vi "Convert Package Display Name (VIPM to NIPM).vi"(8 "error in (no error)":errorcluster, 9 "LabVIEW version in":string, 11 "VIPM Package Display Name":string) -> (0 "error out":errorcluster, 1 "LabVIEW version out":string, 3 "NIPM Package Display Name":string)   [LabVIEW 2014, in "vipm-to-nipm-package-converter.lvlib"]
doc: "Converts the VIPM package's Display Name to a LabVIEW-version specific NIPM Package Display Name. For example, \"OpenG String Library\" and \"18.0\" converts to \"OpenG String Library (LabVIEW 2018 32-bit)\".\n\nINPUT(S):\n<b>LabVIEW version</b>: Specifies the LabVIEW version for the NIPM package to support (\"14.0\", \"14.0 (64-bit)\", \"18.0\", \"18.0 (64-bit)\", etc)"
uses:
  vipm-to-nipm-package-converter.lvlib
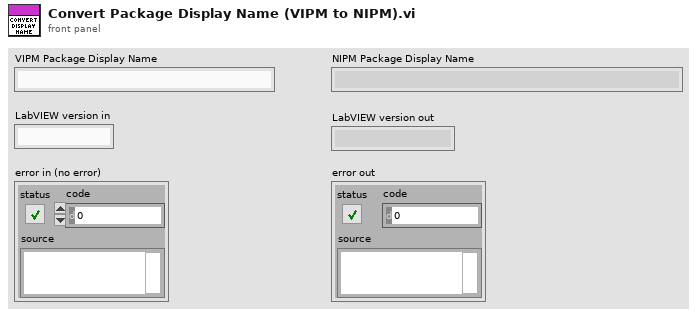
[diagram p1: front panel]
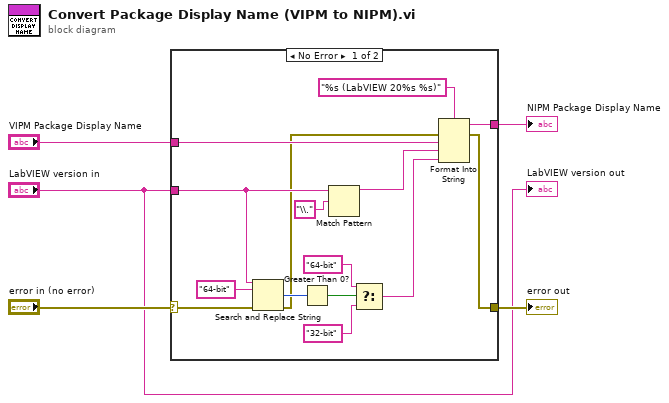
[diagram p0: block diagram]
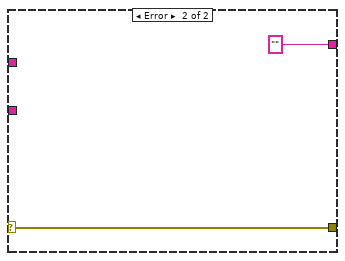
[diagram p2: hidden frame]
diagram:
  n1 = case shown="No Error" "error in (no error)" {
    selector: "error in (no error)" -> [w7 w22]
    tunnel: [w20 w22] -> w5
    tunnel: [w19 ""] -> w4
    tunnel: "VIPM Package Display Name" -> [w18 _]
    tunnel: "LabVIEW version in" -> [w9 _]
    frame No Error {
      n2 = Search and Replace String(input string=w9, search string="64-bit", error in=w7) -> (number of replacements=w15:i32, error out=w6:errorcluster)  [unwired: 5 in, 2 out]
      n3 = Greater Than 0?(x=w15) -> (x > 0?=w14:bool)
      n4 = Match Pattern(string=w9, regular expression="\\.") -> (before substring=w8:string)  [unwired: 1 in, 3 out]
      n5 = Select(t="64-bit" ("search string"), s=w14, f="32-bit" ("search string")) -> (s? t:f=w11:string)
      n6 = Format Into String(format string="%s (LabVIEW 20%s %s)", error in=w6, w18, w8, w11) -> (resulting string=w19:string, error out=w20:errorcluster)  [unwired: 1 in]
    }
    frame Error {
    }
  }
  "error out" <- w5
  "NIPM Package Display Name" <- w4
  "LabVIEW version out" <- "LabVIEW version in"
